vi "MCListbox Event - Key Down.vi"(5 "VKey":T1, 7 "Char":i16, 8 "Error In":errorcluster, 11 "CtlRef":refnum<vi>) -> (0 "Error Out":errorcluster, 2 "Edit Position B4 <RETURN>":cluster{"row":i32, "col":i32})   [LabVIEW 2013]
uses:
  <vilib>/event_ctls.llb/eventvkey.ctl
  <vilib>/Utility/miscctls.llb/LVRowAndColumnTypeDef.ctl
panel:
  out "Blank String":bool
  out "col":i32
  out "row":i32
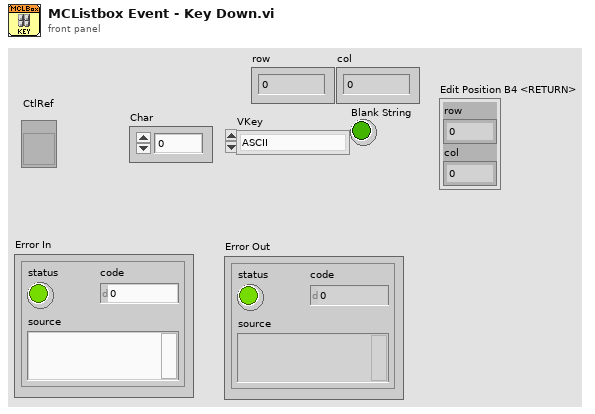
[diagram p1: front panel]
types:
  T1 = typedef "eventvkey.ctl" = enum16{"ASCII", "Enter", "Return", "Shift", "Ctrl", "Alt", "Cmd", "Opt", "Caps", "NumLock", "Clear", "Break", "Up", "Down", "Left", "Right", "Insert", "Delete", "Home", "End", "PageUp", "PageDown", "Escape", "Help", "Pause", "ScrollLock", "F1", "F2", "F3", "F4", "F5", "F6", "F7", "F8", "F9", "F10", "F11", "F12", "F13", "F14", "F15", "F16", "F17", "F18", "F19", "F20", "F21", "F22", "F23", "F24", "Play", "VolumeUp", "VolumeDown", "Mute", "Two Byte Char"}
  T2 = typedef "LVRowAndColumnTypeDef.ctl" = cluster{"Row":i32, "Column":i32}
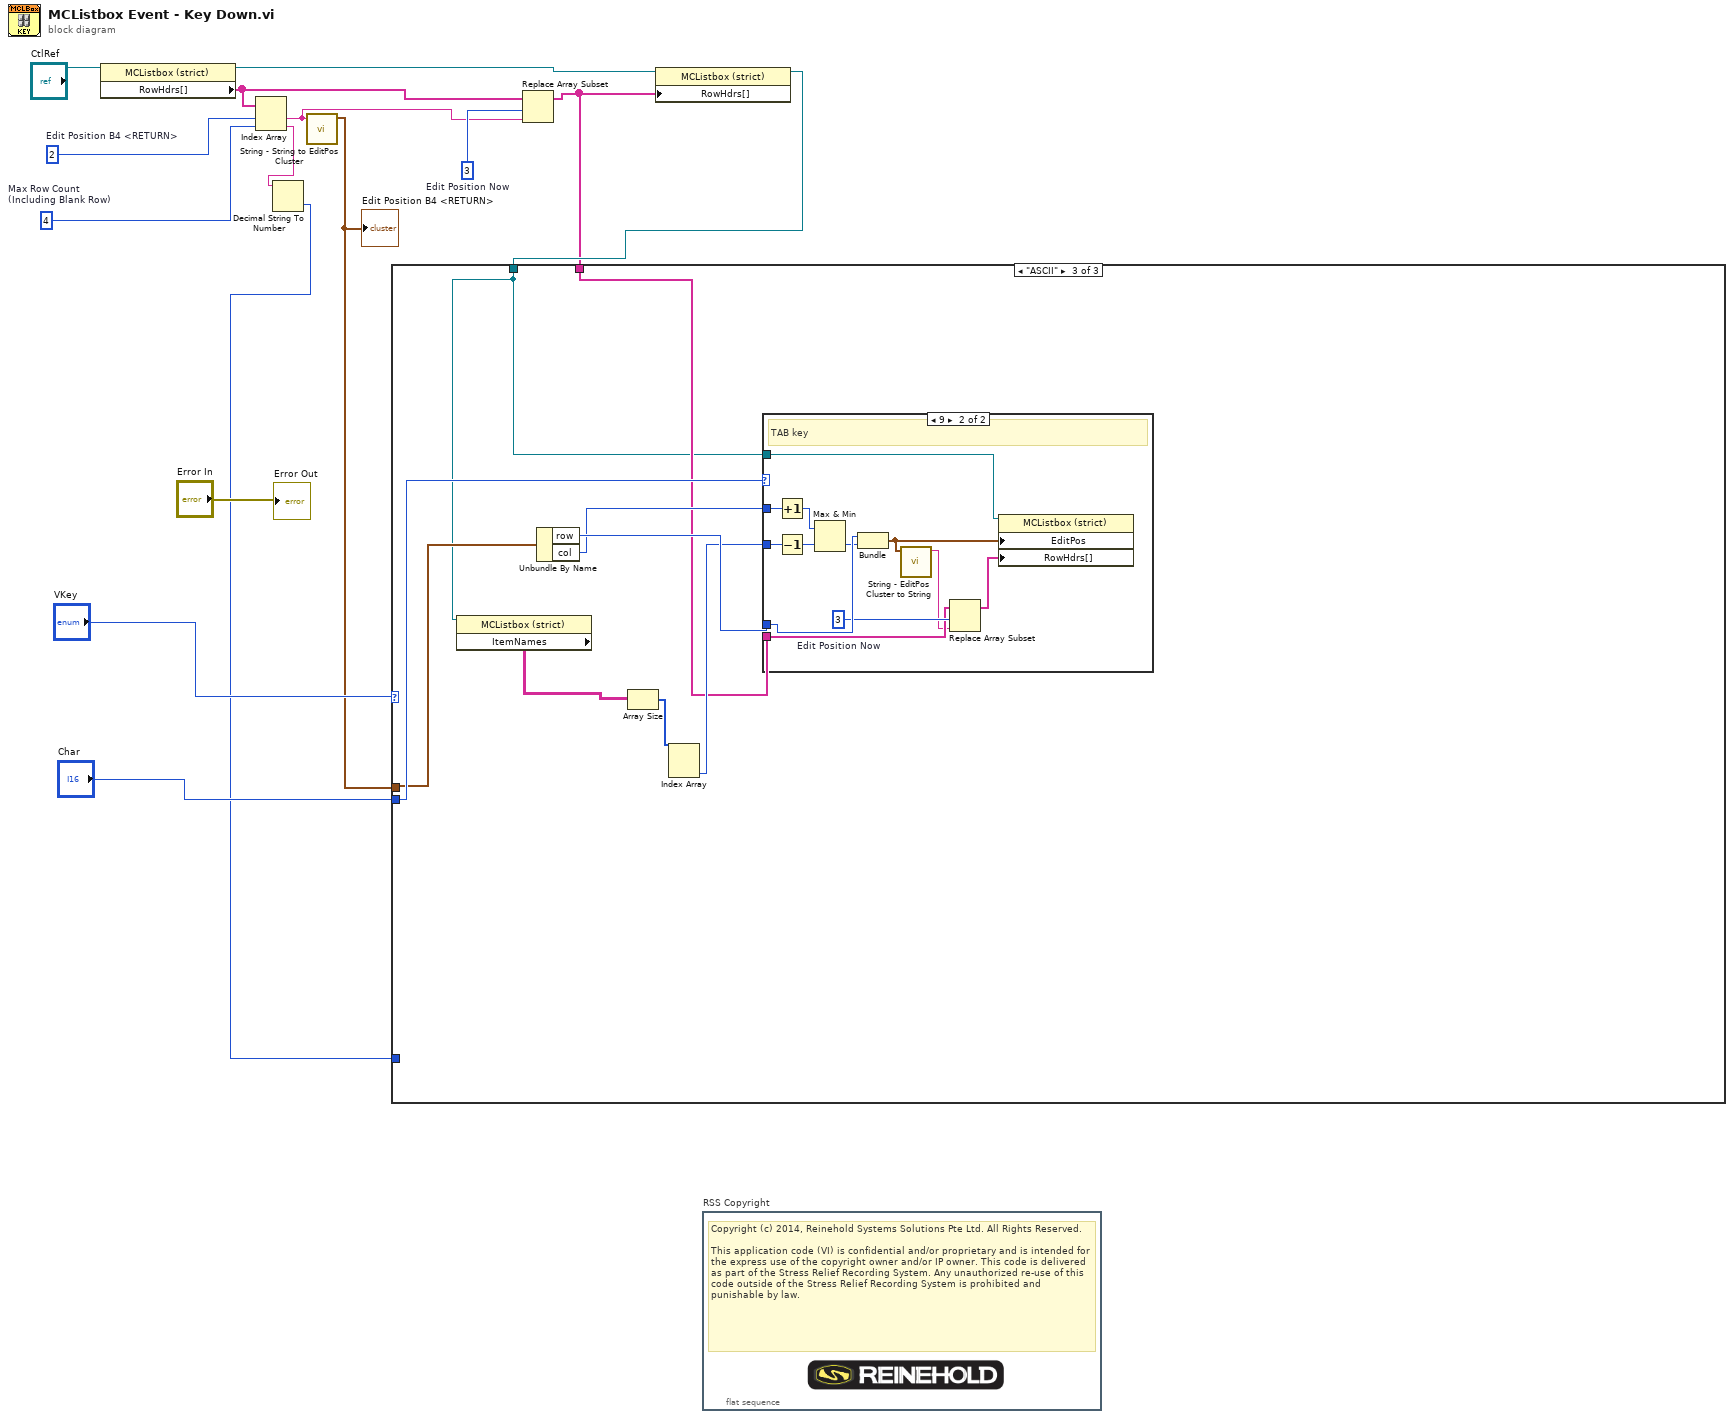
[diagram p0: block diagram]
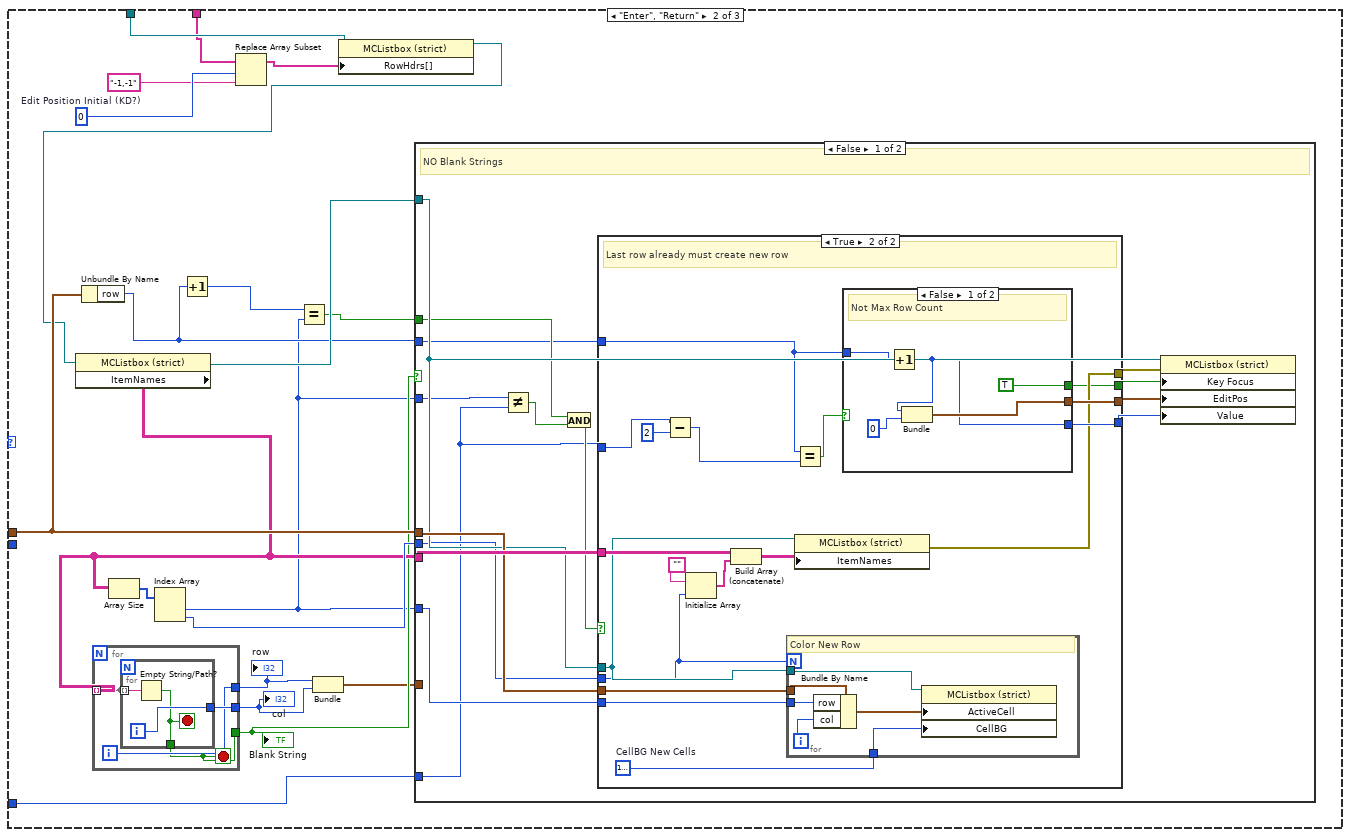
[diagram p3: hidden frame]
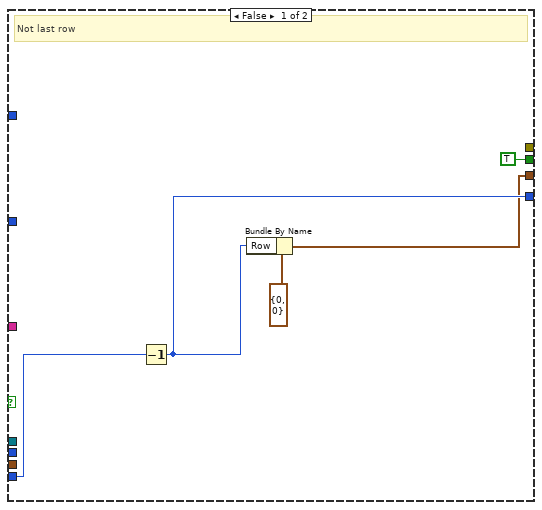
[diagram p4: hidden frame]
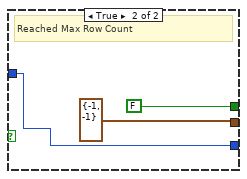
[diagram p5: hidden frame]
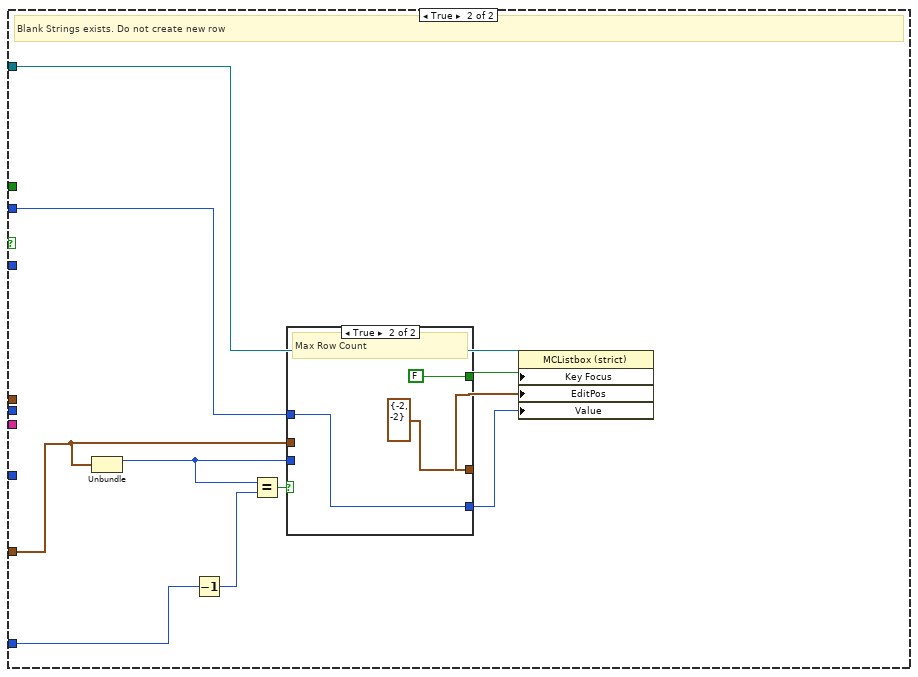
[diagram p6: hidden frame]
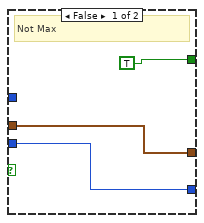
[diagram p7: hidden frame]
diagram:
  w2 = 4  # Max Row Count (Including Blank Row)
  w10 = 3  # Edit Position Now
  w13 = 2  # Edit Position B4 <RETURN>
  n1 = property on="Property Node" class="MCListbox (strict)"(reference="CtlRef") -> (reference out=w12:refnum<vi>, "RowHdrs[]"=w11:string[])  [unwired: 1 in, 1 out]
  n2 = Index Array(array=w11, index #1=w13, index #2=w2) -> (element #1=w6:string, element #2=w3:string)
  n3 = Decimal String To Number(string=w3) -> (number=w1:i32)  [unwired: 2 in, 1 out]
  n4 = call "String - String to EditPos Cluster.vi"("string"=w6) -> ("EditPos"=w5:cluster{"row":i32, "col":i32})  [unwired: 10 in]
  "Edit Position B4 <RETURN>" <- w5
  n5 = Replace Array Subset(array=w11, new element=w6, index=w10) -> (w7:string[])
  n6 = property on="Property Node" class="MCListbox (strict)"(reference=w12, "RowHdrs[]"=w7) -> (reference out=w8:refnum<vi>)  [unwired: 1 in, 1 out]
  n7 = case shown="\"ASCII\"" "VKey" {
    tunnel: w5 -> [_ w30 w118]
    tunnel: "Char" -> [_ _ w119]
    tunnel: w8 -> [_ w28 w111]
    tunnel: w7 -> [_ w27 w112]
    tunnel: w1 -> [_ w16 _]
    frame Default {
    }
    frame "Enter", "Return" {
      w26 = 0  # Edit Position Initial (KD?)
      n8 = Unbundle By Name(w30) -> ("row"=w29:i32)
      n9 = Increment(x=w29) -> (x+1=w32:i32)
      n10 = Replace Array Subset(array=w27, new element="-1,-1" ("new element/subarray"), index=w26) -> (w24:string[])
      n11 = property on="Property Node" class="MCListbox (strict)"(reference=w28, "RowHdrs[]"=w24) -> (reference out=w23:refnum<vi>)  [unwired: 1 in, 1 out]
      n12 = property on="Property Node" class="MCListbox (strict)"(reference=w23) -> (reference out=w35:refnum<vi>, "ItemNames"=w22:string[][])  [unwired: 1 in, 1 out]
      n13 = for {
        tunnel: [w39] -> _ mode=indexing
        tunnel: w22 -> [w39] mode=indexing
        tunnel: [w38] -> w19
        tunnel: [w37] -> w20
        tunnel: [w36] -> w21
        i -> [w37]
        stop <- w36 stop-if-true
        n14 = for {
          tunnel: w39 -> [w42] mode=indexing
          tunnel: [w40] -> w36
          tunnel: [w41] -> w38
          i -> [w41]
          stop <- w40 stop-if-true
          n15 = Empty String/Path?(string/path=w42) -> (empty?=w40:bool)
        }
      }
      "row" <- w20
      "col" <- w19
      "Blank String" <- w21
      n16 = Array Size(array=w22) -> (size(s)=w34:i32[])
      n17 = Index Array(array=w34) -> (element #1=w17:i32, element #2=w33:i32)  [unwired: 2 in]
      n18 = Equal?(x=w32, y=w17) -> (x = y?=w31:bool)
      n19 = Bundle(w20, w19) -> (w18:cluster{i32, i32})  [unwired: 1 in]
      n20 = case shown="False" w21 {
        tunnel: w30 -> [w56 _]
        tunnel: w22 -> [w57 _]
        tunnel: w29 -> [w44 w95]
        tunnel: w35 -> [w55 w104]
        tunnel: w33 -> [w54 _]
        tunnel: w31 -> [w46 _]
        tunnel: w17 -> [w52 _]
        tunnel: w18 -> [_ w100]
        tunnel: w16 -> [w43 w98]
        tunnel: w17 -> [w47 _]
        frame False {
          # "NO Blank Strings"
          n21 = Not Equal?(x=w47, y=w43) -> (x != y?=w45:bool)
          n22 = And(x=w46, y=w45) -> (x .and. y?=w48:bool)
          n23 = case shown="True" w48 {
            tunnel: w57 -> [_ w80]
            tunnel: w56 -> [_ w79]
            tunnel: w55 -> [_ w78]
            tunnel: w54 -> [_ w75]
            tunnel: w52 -> [w62 w65]
            tunnel: [_ w69] -> w53
            tunnel: [w60 w71] -> w51
            tunnel: [w59 w70] -> w50
            tunnel: [TRUE w68] -> w49
            tunnel: w43 -> [_ w67]
            tunnel: w44 -> [_ w64]
            frame False {
              # "Not last row"
              n24 = Decrement(x=w62) -> (x-1=w60:i32)
              n25 = Bundle By Name(cluster=T2 {"Row"=0, "Column"=0} ("Row-Col Cluster Out"), "Row"=w60) -> (w59:T2)
            }
            frame True {
              w73 = u32 16777225  # CellBG New Cells
              # "Last row already must create new row"
              n26 = Subtract(x=w67, y=2) -> (x-y=w63:i32)
              n27 = Initialize Array("", w75) -> (w74:string[])
              n28 = Build Array (concatenate)(w80, w74) -> (w77:string[][])
              n29 = for {
                N: w75 -> [_]
                tunnel: w65 -> [w94]
                tunnel: w79 -> [w92]
                tunnel: w73 -> [w90]
                tunnel: w78 -> [w89]
                i -> [w91]
                # "Color New Row"
                n30 = Bundle By Name(cluster=w92, "row"=w94, "col"=w91) -> (w93:cluster{"row":i32, "col":i32})
                n31 = property on="Property Node" class="MCListbox (strict)"(reference=w89, "ActiveCell"=w93, "CellBG"=w90) -> ()  [unwired: 1 in, 2 out]
              }
              n32 = Equal?(x=w64, y=w63) -> (x = y?=w72:bool)
              n33 = property on="Property Node" class="MCListbox (strict)"(reference=w78, "ItemNames"=w77) -> (error out=w69:errorcluster)  [unwired: 1 in, 1 out]
              n34 = case shown="False" w72 {
                tunnel: [w81 w86] -> w71
                tunnel: [w85 T2 {"Row"=-1, "Column"=-1} ("Row-Col Cluster Out")] -> w70
                tunnel: [TRUE FALSE] -> w68
                tunnel: w64 -> [w82 w86]
                frame False {
                  # "Not Max Row Count"
                  n35 = Increment(x=w82) -> (x+1=w81:i32)
                  n36 = Bundle(w81, 0) -> (w85:cluster{i32, i32})  [unwired: 1 in]
                }
                frame True {
                  # "Reached Max Row Count"
                }
              }
            }
          }
          n37 = property on="Property Node" class="MCListbox (strict)"(reference=w55, error in=w53, "Key Focus"=w49, "EditPos"=w50, "Value"=w51) -> ()  [unwired: 2 out]
        }
        frame True {
          # "Blank Strings exists. Do not create new row"
          n38 = Unbundle(w100) -> (w101:i32)  [unwired: 1 out]
          n39 = Decrement(x=w98) -> (x-1=w103:i32)
          n40 = Equal?(x=w101, y=w103) -> (x = y?=w102:bool)
          n41 = case shown="True" w102 {
            tunnel: w101 -> [w107 _]
            tunnel: w100 -> [w106 _]
            tunnel: [w106 cluster{i32, i32} {-2, -2}] -> w99
            tunnel: [w107 w108] -> w97
            tunnel: [TRUE ("Key Focus") FALSE ("Key Focus")] -> w96
            tunnel: w95 -> [_ w108]
            frame False {
              # "Not Max"
            }
            frame True {
              # "Max Row Count"
            }
          }
          n42 = property on="Property Node" class="MCListbox (strict)"(reference=w104, "Key Focus"=w96, "EditPos"=w99, "Value"=w97) -> ()  [unwired: 1 in, 2 out]
        }
      }
    }
    frame "ASCII" {
      n43 = property on="Property Node" class="MCListbox (strict)"(reference=w111) -> ("ItemNames"=w115:string[][])  [unwired: 1 in, 2 out]
      n44 = Unbundle By Name(w118) -> ("row"=w117:i32, "col"=w116:i32)
      n45 = Array Size(array=w115) -> (size(s)=w114:i32[])
      n46 = Index Array(array=w114) -> (element #2=w113:i32)  [unwired: 2 in, 1 out]
      n47 = case shown="9" w119 {
        tunnel: w117 -> [_ w131]
        tunnel: w116 -> [_ w128]
        tunnel: w113 -> [_ w130]
        tunnel: w111 -> [_ w125]
        tunnel: w112 -> [_ w123]
        frame 0, Default {
        }
        frame 9 {
          w124 = 3  # Edit Position Now
          # "TAB key"
          n48 = Increment(x=w128) -> (x+1=w127:i32)
          n49 = Decrement(x=w130) -> (x-1=w129:i32)
          n50 = Max & Min(x=w127, y=w129) -> (min(x,y)=w126:i32)  [unwired: 1 out]
          n51 = Bundle("row"=w131, w126) -> (w121:cluster{"row":i32, i32})  [unwired: 1 in]
          n52 = call "String - EditPos Cluster to String.vi"("EditPos"=w121) -> ("result string"=w120:string)  [unwired: 10 in]
          n53 = Replace Array Subset(array=w123, new element=w120, index=w124) -> (w122:string[])
          n54 = property on="Property Node" class="MCListbox (strict)"(reference=w125, "EditPos"=w121, "RowHdrs[]"=w122) -> ()  [unwired: 1 in, 2 out]
        }
      }
    }
  }
  n55 = flat-sequence "RSS Copyright" {
    frame #0 {
      # "Copyright (c) 2014, Reinehold Systems Solutions Pte Ltd. All Rights Reserved.\n\nThis application code (VI) is confidential and/or proprietary and is intended for the express use of the copyright owner and/or IP owner. This code is delivered as part of the Stress Relief Recording System. Any unauthorized re-use of this code outside of the Stress Relief Recording System is prohibited and punishable by law."
    }
  }
  "Error Out" <- "Error In"
